vi "CAL_GCP_R_EXT.vi"(0 "R_ROLL":sgl, 5 "Acc_Z":sgl, 9 "Param_In":T1) -> (4 "R_NUM":u32, 6 "R_Ctrl_Start":bool, 8 "R_RUN_OK":bool, 10 "R_GCP_EXT":sgl, 14 "R_GCP_Total_Time":sgl, 15 "R_Period":u32)   [LabVIEW 2019]
uses:
  RT_GLOBAL.vi
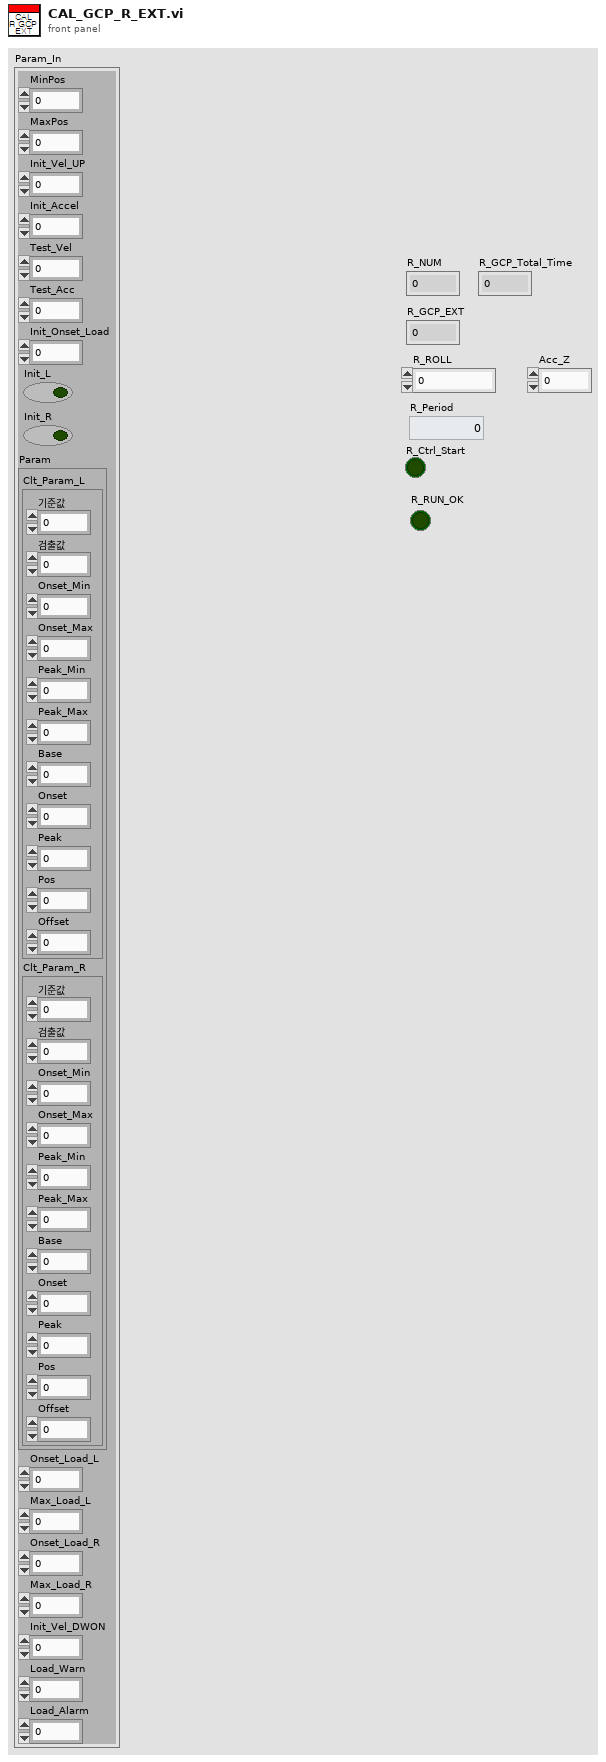
[diagram p1: front panel]
types:
  T1 = cluster{"MinPos":i32, "MaxPos":i32, "Init_Vel_UP":i32, "Init_Accel":u32, "Test_Vel":i32, "Test_Acc":u32, "Init_Onset_Load":sgl, "Init_L":bool, "Init_R":bool, "Param":cluster{"Clt_Param_L":cluster{"기준값":sgl, "검출값":sgl, "Onset_Min":sgl, "Onset_Max":sgl, "Peak_Min":sgl, "Peak_Max":sgl, "Base":i32, "Onset":i32, "Peak":i32, "Pos":i32, "Offset":sgl}, "Clt_Param_R":cluster{"기준값":sgl, "검출값":sgl, "Onset_Min":sgl, "Onset_Max":sgl, "Peak_Min":sgl, "Peak_Max":sgl, "Base":i32, "Onset":i32, "Peak":i32, "Pos":i32, "Offset":sgl}}, "Onset_Load_L":sgl, "Max_Load_L":sgl, "Onset_Load_R":sgl, "Max_Load_R":sgl, "Init_Vel_DWON":i32, "Load_Warn":sgl, "Load_Alarm":sgl}
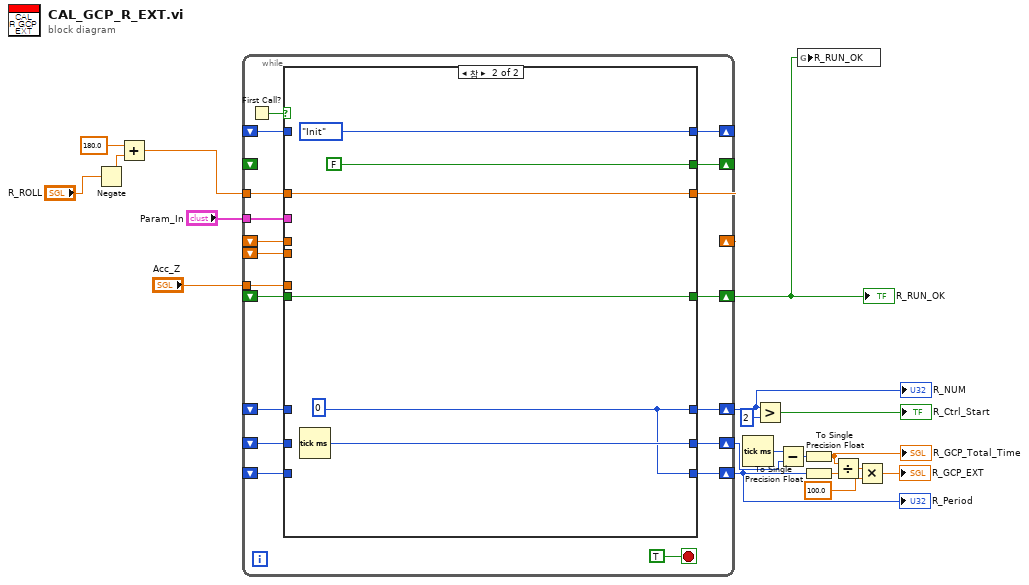
[diagram p0: block diagram]
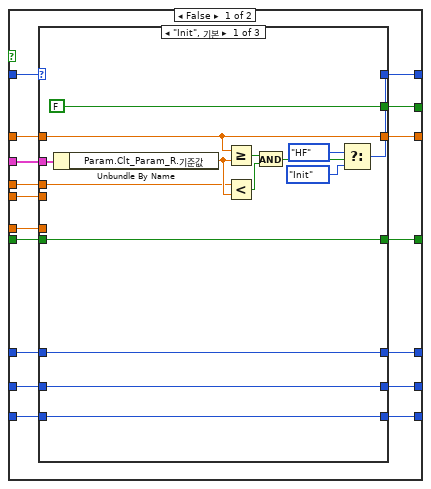
[diagram p2: hidden frame]
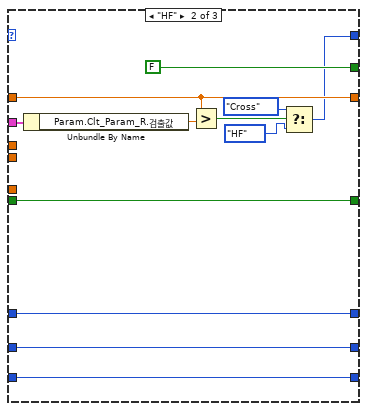
[diagram p3: hidden frame]
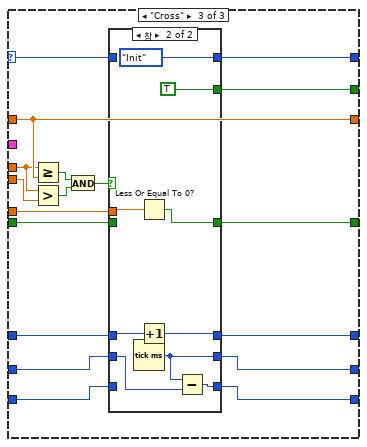
[diagram p4: hidden frame]
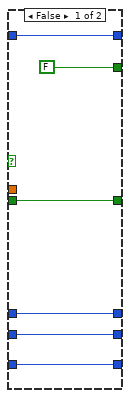
[diagram p5: hidden frame]
diagram:
  n1 = Negate(x="R_ROLL") -> (-x=w7:sgl)
  n2 = Add(x=sgl 180.0, y=w7) -> (x+y=w5:sgl)
  n3 = while {
    tunnel: w5 -> [w32]
    tunnel: "Param_In" -> [w25]
    shift-right: [w35] -> _
    shift-left: _ -> [w36]
    shift-right: [w34] -> _
    shift-left: _ -> [_]
    shift-right: [w33] -> _
    shift-left: _ -> [w24]
    shift-left: _ -> [w23]
    shift-right: [w30] -> w19
    shift-left: _ -> [w31]
    shift-right: [w29] -> w11
    shift-left: _ -> [w26]
    shift-right: [w28] -> w9
    shift-left: _ -> [w27]
    shift-right: [w21] -> w1
    shift-left: _ -> [w22]
    tunnel: "Acc_Z" -> [w20]
    stop <- TRUE stop-if-true
    n4 = First Call?() -> (First Call?: T/F=w37:bool)
    n5 = case shown="참" w37 {
      tunnel: w36 -> [w55 _]
      tunnel: [w50 enum16{"Init", "HF", "Cross"}."Init"] -> w35
      tunnel: [w51 FALSE] -> w34
      tunnel: [w52 w119] -> w33
      tunnel: w32 -> [w53 w119]
      tunnel: w31 -> [w48 _]
      tunnel: [w49 w117] -> w30
      tunnel: [w46 w118] -> w29
      tunnel: [w45 w117] -> w28
      tunnel: w27 -> [w44 _]
      tunnel: w26 -> [w47 _]
      tunnel: w25 -> [w54 _]
      tunnel: w24 -> [w43 _]
      tunnel: w23 -> [w42 _]
      tunnel: w22 -> [w41 w116]
      tunnel: [w40 w116] -> w21
      tunnel: w20 -> [w39 _]
      frame False {
        n6 = case shown="\"Init\", 기본" w55 {
          selector: w55 -> [_ _ w100]
          tunnel: w54 -> [w63 w82 _]
          tunnel: w53 -> [w61 w77 w97]
          tunnel: [w61 w77 w97] -> w52
          tunnel: [FALSE FALSE w98] -> w51
          tunnel: [w60 w75 w99] -> w50
          tunnel: [w59 w74 w90] -> w49
          tunnel: w48 -> [w59 w74 w91]
          tunnel: w47 -> [w58 w73 w89]
          tunnel: [w58 w73 w87] -> w46
          tunnel: [w57 w72 w86] -> w45
          tunnel: w44 -> [w57 w72 w88]
          tunnel: w43 -> [w62 _ w96]
          tunnel: w42 -> [_ _ w95]
          tunnel: w41 -> [w56 w71 w85]
          tunnel: [w56 w71 w84] -> w40
          tunnel: w39 -> [_ _ w83]
          frame "Init", Default {
            n7 = Unbundle By Name(w63) -> ("Param.Clt_Param_R.기준값"=w64:sgl)
            n8 = Greater Or Equal?(x=w61, y=w64) -> (x >= y?=w69:bool)
            n9 = Less?(x=w62, y=w64) -> (x < y?=w68:bool)
            n10 = And(x=w69, y=w68) -> (x .and. y?=w67:bool)
            n11 = Select(t=enum16{"Init", "HF", "Cross"}."HF", s=w67, f=enum16{"Init", "HF", "Cross"}."Init") -> (s? t:f=w60:enum16{"Init", "HF", "Cross"})
          }
          frame "HF" {
            n12 = Unbundle By Name(w82) -> ("Param.Clt_Param_R.검출값"=w78:sgl)
            n13 = Greater?(x=w77, y=w78) -> (0:w79:bool)
            n14 = Select(t=enum16{"Init", "HF", "Cross"}."Cross", s=w79, f=enum16{"Init", "HF", "Cross"}."HF") -> (s? t:f=w75:enum16{"Init", "HF", "Cross"})
          }
          frame "Cross" {
            n15 = Greater Or Equal?(x=w96, y=w97) -> (x >= y?=w94:bool)
            n16 = Greater?(x=w96, y=w95) -> (0:w93:bool)
            n17 = And(x=w94, y=w93) -> (x .and. y?=w92:bool)
            n18 = case shown="참" w92 {
              tunnel: w100 -> [w102 _]
              tunnel: [w102 enum16{"Init", "HF", "Cross"}."Init"] -> w99
              tunnel: [FALSE TRUE] -> w98
              tunnel: w91 -> [w104 w113]
              tunnel: [w104 w112] -> w90
              tunnel: w89 -> [w105 w111]
              tunnel: w88 -> [w106 _]
              tunnel: [w106 w110] -> w86
              tunnel: [w105 w109] -> w87
              tunnel: w85 -> [w101 _]
              tunnel: [w101 w107] -> w84
              tunnel: w83 -> [_ w108]
              frame False {
              }
              frame True {
                n19 = Tick Count (ms)() -> (millisecond timer value=w109:u32)
                n20 = Less Or Equal To 0?(x=w108) -> (x <= 0?=w107:bool)
                n21 = Increment(x=w113) -> (x+1=w112:u32)
                n22 = Subtract(x=w109, y=w111) -> (x-y=w110:u32)
              }
            }
          }
        }
      }
      frame True {
        w117 = u32 0
        n23 = Tick Count (ms)() -> (millisecond timer value=w118:u32)
      }
    }
  }
  "R_NUM" <- w19
  "R_Period" <- w9
  "R_RUN_OK" <- w1
  n24 = Tick Count (ms)() -> (millisecond timer value=w13:u32)
  n25 = Greater?(x=w19, y=u32 2) -> (0:→"R_Ctrl_Start":bool)
  n26 = Subtract(x=w13, y=w11) -> (x-y=w12:u32)
  n27 = global write "RT_GLOBAL.vi" "R_RUN_OK"(w1) -> ()
  n28 = To Single Precision Float(number=w12) -> (single precision float=w8:sgl)
  "R_GCP_Total_Time" <- w8
  n29 = To Single Precision Float(number=w9) -> (single precision float=w16:sgl)
  n30 = Divide(x=w8, y=w16) -> (x/y=w15:sgl)
  n31 = Multiply(x=w15, y=sgl 100.0) -> (x*y=→"R_GCP_EXT":sgl)
